vi "Report Error.vi"(8 "error in (no error)":errorcluster, 11 "Self Enqueuer":refnum<class "Message Enqueuer.lvclass">) -> (0 "error out":errorcluster)   [LabVIEW 2016, in "Assert API Components.lvlib" / "Base UI Actor.lvlib" / "Base UI Actor.lvclass"]
uses:
  Base UI Actor.lvclass
  <vilib>/ActorFramework/Message Enqueuer/Message Enqueuer.lvclass
  <vilib>/ActorFramework/Report Error Msg/Report Error Msg.lvclass/Report Error Msg.ctl
  <vilib>/ActorFramework/Message Enqueuer/Message Enqueuer.lvclass/Message Enqueuer.ctl
  <vilib>/ActorFramework/Message Enqueuer/Enqueue.vi
  <vilib>/ActorFramework/Report Error Msg/Report Error Msg.lvclass
  C:/Program Files (x86)/National Instruments/LabVIEW 2016/vi.lib/ActorFramework/Message/Message.lvclass
  <vilib>/Utility/LVClass/Get LV Class Name.vi
  <resource>/AFDebug/Generate Trace for Message.vi
  <vilib>/ActorFramework/Message Priority Queue/Priority Enqueue.vi
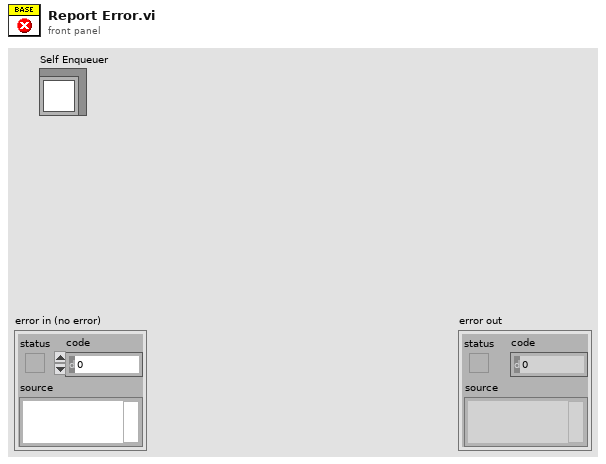
[diagram p1: front panel]
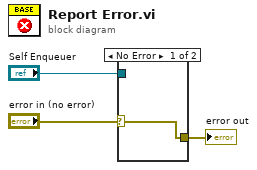
[diagram p0: block diagram]
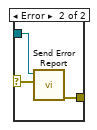
[diagram p2: hidden frame]
diagram:
  n1 = case shown="No Error" "error in (no error)" {
    selector: "error in (no error)" -> [w4 w7]
    tunnel: "Self Enqueuer" -> [_ w6]
    tunnel: [w4 w5] -> w1
    frame No Error {
    }
    frame Error {
      n2 = call <vilib>:"Send Error Report.vi"("Error From Sender"=w7, "Message Enqueuer"=w6) -> ("error out"=w5:errorcluster)  [unwired: 9 in]
    }
  }
  "error out" <- w1
